vi "2 station_keeping_points.vi"(9 "Which Point?":i32, 10 "Midpoint":T1 {"North" format="%#_10f"; "East" format="%#_8f"}) -> (2 "Waypoint":T1 {"North" format="%#_10f"; "East" format="%#_8f"})   [LabVIEW 2011]
doc: "The station keeping mission steps through a series of waypoints from 1 : n. This takes which point it is on, and returns the coordinates. It uses modular arithmetic to cycle through a set of waypoints. The waypoints are shifted upwind, and usually oriented with respect to the wind somehow."
uses:
  2 Typedefs/UTM Location.ctl
  2 Typedefs/absolute wind direction.ctl
  2 Globals/2 Global.vi
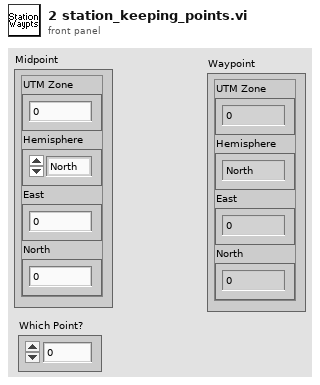
[diagram p1: front panel]
types:
  T1 = typedef "UTM Location.ctl" = cluster{"UTM Zone":i32, "Hemisphere":enum16{"North", "South"}, "East":dbl, "North":dbl}
  T2 = typedef "absolute wind direction.ctl" = dbl
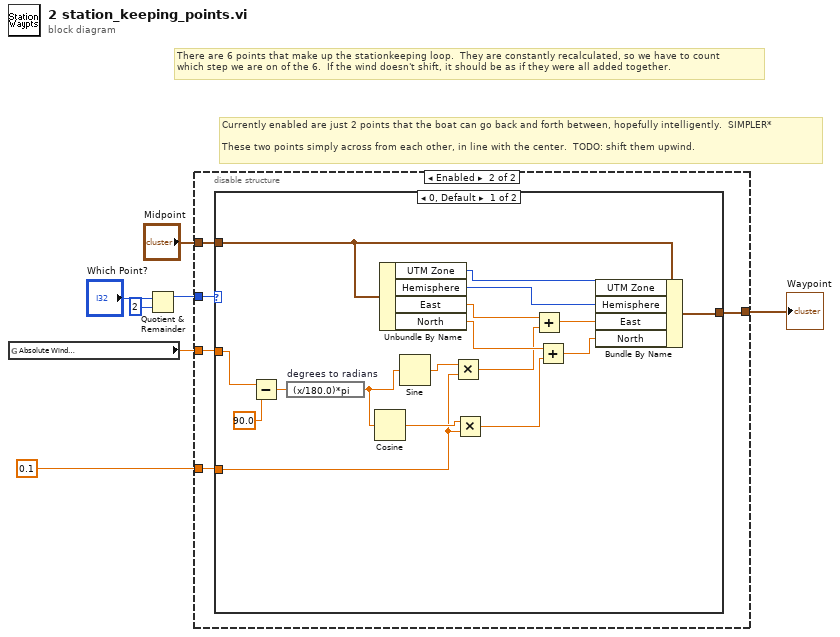
[diagram p0: block diagram]
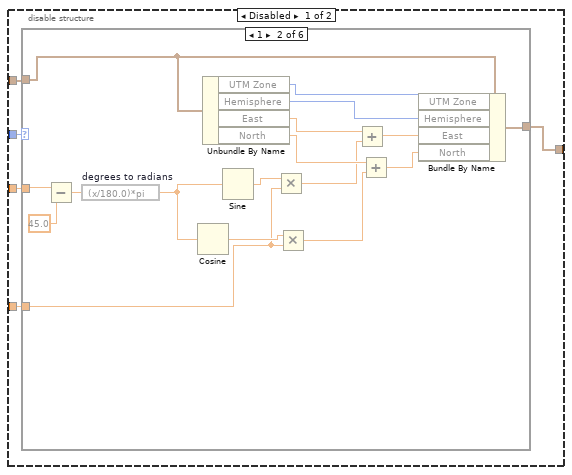
[diagram p2: hidden frame]
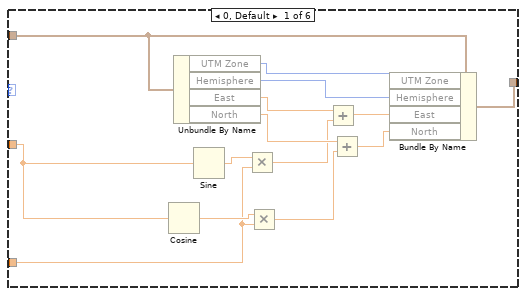
[diagram p3: hidden frame]
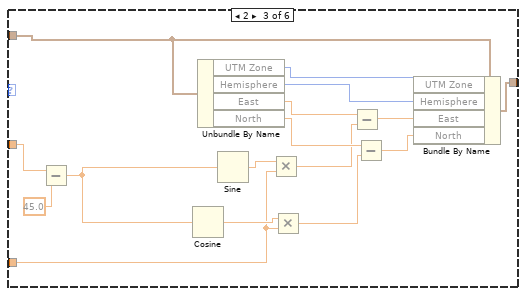
[diagram p4: hidden frame]
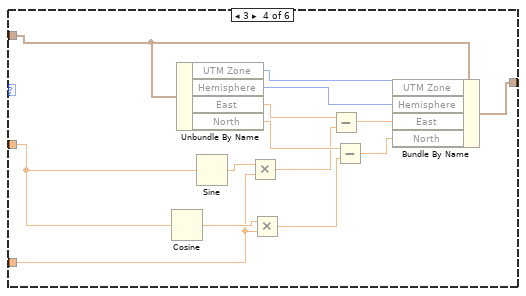
[diagram p5: hidden frame]
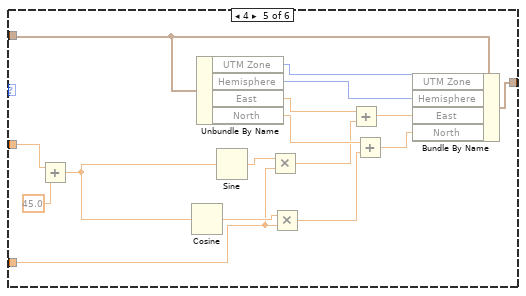
[diagram p6: hidden frame]
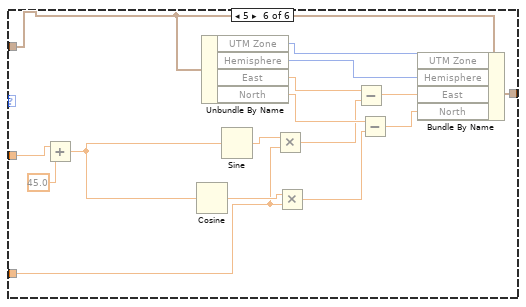
[diagram p7: hidden frame]
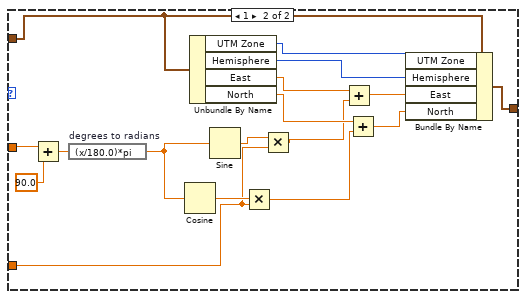
[diagram p8: hidden frame]
diagram:
  # "Currently enabled are just 2 points that the boat can go back and forth between, hopefully intelligently.  SIMPLER*\n\nThese two points simply across from each other, in line with the center.  TODO: shift them upwind."
  # "There are 6 points that make up the stationkeeping loop.  They are constantly recalculated, so we have to count\nwhich step we are on of the 6.  If the wind doesn't shift, it should be as if they were all added together."
  n1 = global read "2 Global.vi" "Absolute Wind\nDirection (º)"() -> (w3:T2)
  n2 = Quotient & Remainder(x="Which Point?", y=2) -> (x-y*floor(x/y)=w5:i32)  [unwired: 1 out]
  n3 = disable-structure shown="Enabled" {
    disable-tunnel: w5 -> [w12 w110]
    disable-tunnel: "Midpoint" -> [w11 w109]
    disable-tunnel: w3 -> [w10 w108]
    disable-tunnel: [w9 w106] -> w2
    disable-tunnel: T2 0.1 ("y") -> [w8 w107]
    frame Disabled {
      n4 = case shown="1" w12 {
        tunnel: w11 -> [w25 w32 w46 w62 w76 w92]
        tunnel: w10 -> [w14 w31 w45 w61 w75 w91]
        tunnel: [w26 w33 w47 w63 w77 w93] -> w9
        tunnel: w8 -> [w13 w29 w44 w60 w74 w90]
        frame 0, Default {
          n5 = Cosine(x=w14) -> (cos(x)=w21:T2)
          n6 = Unbundle By Name(w25) -> ("UTM Zone"=w24:i32, "Hemisphere"=w23:enum16{"North", "South"}, "East"=w19:dbl, "North"=w17:dbl)
          n7 = Sine(x=w14) -> (sin(x)=w22:T2)
          n8 = Multiply(x=w22, y=w13) -> (x*y=w16:T2)
          n9 = Multiply(x=w21, y=w13) -> (x*y=w15:T2)
          n10 = Add(x=w19, y=w16) -> (x+y=w20:T2)
          n11 = Add(x=w17, y=w15) -> (x+y=w18:T2)
          n12 = Bundle By Name(cluster=w25, "UTM Zone"=w24, "Hemisphere"=w23, "East"=w20, "North"=w18) -> (w26:T1)
        }
        frame 1 {
          n13 = Subtract(x=w31, y=T2 45.0) -> (x-y=w28:T2)
          n14 = expression code="(x/180.0)*pi" "degrees to radians"(w28) -> (w27:T2)
          n15 = Cosine(x=w27) -> (cos(x)=w40:T2)
          n16 = Unbundle By Name(w32) -> ("UTM Zone"=w43:i32, "Hemisphere"=w42:enum16{"North", "South"}, "East"=w38:dbl, "North"=w36:dbl)
          n17 = Sine(x=w27) -> (sin(x)=w41:T2)
          n18 = Multiply(x=w41, y=w29) -> (x*y=w35:T2)
          n19 = Multiply(x=w40, y=w29) -> (x*y=w34:T2)
          n20 = Add(x=w38, y=w35) -> (x+y=w39:T2)
          n21 = Add(x=w36, y=w34) -> (x+y=w37:T2)
          n22 = Bundle By Name(cluster=w32, "UTM Zone"=w43, "Hemisphere"=w42, "East"=w39, "North"=w37) -> (w33:T1)
        }
        frame 2 {
          n23 = Subtract(x=w45, y=T2 45.0) -> (x-y=w49:T2)
          n24 = Cosine(x=w49) -> (cos(x)=w56:T2)
          n25 = Unbundle By Name(w46) -> ("UTM Zone"=w59:i32, "Hemisphere"=w58:enum16{"North", "South"}, "East"=w54:dbl, "North"=w52:dbl)
          n26 = Sine(x=w49) -> (sin(x)=w57:T2)
          n27 = Multiply(x=w57, y=w44) -> (x*y=w51:T2)
          n28 = Multiply(x=w56, y=w44) -> (x*y=w50:T2)
          n29 = Subtract(x=w54, y=w51) -> (x-y=w55:T2)
          n30 = Subtract(x=w52, y=w50) -> (x-y=w53:T2)
          n31 = Bundle By Name(cluster=w46, "UTM Zone"=w59, "Hemisphere"=w58, "East"=w55, "North"=w53) -> (w47:T1)
        }
        frame 3 {
          n32 = Cosine(x=w61) -> (cos(x)=w70:T2)
          n33 = Unbundle By Name(w62) -> ("UTM Zone"=w73:i32, "Hemisphere"=w72:enum16{"North", "South"}, "East"=w68:dbl, "North"=w66:dbl)
          n34 = Sine(x=w61) -> (sin(x)=w71:T2)
          n35 = Multiply(x=w71, y=w60) -> (x*y=w65:T2)
          n36 = Multiply(x=w70, y=w60) -> (x*y=w64:T2)
          n37 = Subtract(x=w68, y=w65) -> (x-y=w69:T2)
          n38 = Subtract(x=w66, y=w64) -> (x-y=w67:T2)
          n39 = Bundle By Name(cluster=w62, "UTM Zone"=w73, "Hemisphere"=w72, "East"=w69, "North"=w67) -> (w63:T1)
        }
        frame 4 {
          n40 = Add(x=w75, y=T2 45.0) -> (x+y=w79:T2)
          n41 = Cosine(x=w79) -> (cos(x)=w86:T2)
          n42 = Unbundle By Name(w76) -> ("UTM Zone"=w89:i32, "Hemisphere"=w88:enum16{"North", "South"}, "East"=w84:dbl, "North"=w82:dbl)
          n43 = Sine(x=w79) -> (sin(x)=w87:T2)
          n44 = Multiply(x=w87, y=w74) -> (x*y=w81:T2)
          n45 = Multiply(x=w86, y=w74) -> (x*y=w80:T2)
          n46 = Add(x=w84, y=w81) -> (x+y=w85:T2)
          n47 = Add(x=w82, y=w80) -> (x+y=w83:T2)
          n48 = Bundle By Name(cluster=w76, "UTM Zone"=w89, "Hemisphere"=w88, "East"=w85, "North"=w83) -> (w77:T1)
        }
        frame 5 {
          n49 = Add(x=w91, y=T2 45.0) -> (x+y=w95:T2)
          n50 = Cosine(x=w95) -> (cos(x)=w102:T2)
          n51 = Unbundle By Name(w92) -> ("UTM Zone"=w105:i32, "Hemisphere"=w104:enum16{"North", "South"}, "East"=w100:dbl, "North"=w98:dbl)
          n52 = Sine(x=w95) -> (sin(x)=w103:T2)
          n53 = Multiply(x=w103, y=w90) -> (x*y=w97:T2)
          n54 = Multiply(x=w102, y=w90) -> (x*y=w96:T2)
          n55 = Subtract(x=w100, y=w97) -> (x-y=w101:T2)
          n56 = Subtract(x=w98, y=w96) -> (x-y=w99:T2)
          n57 = Bundle By Name(cluster=w92, "UTM Zone"=w105, "Hemisphere"=w104, "East"=w101, "North"=w99) -> (w93:T1)
        }
      }
    }
    frame Enabled {
      n58 = case shown="0, Default" w110 {
        tunnel: w109 -> [w126 w134]
        tunnel: w108 -> [w112 w133]
        tunnel: [w127 w135] -> w106
        tunnel: w107 -> [w115 w131]
        frame 0, Default {
          n59 = Subtract(x=w112, y=T2 90.0) -> (x-y=w113:T2)
          n60 = expression code="(x/180.0)*pi" "degrees to radians"(w113) -> (w111:T2)
          n61 = Cosine(x=w111) -> (cos(x)=w122:T2)
          n62 = Unbundle By Name(w126) -> ("UTM Zone"=w125:i32, "Hemisphere"=w124:enum16{"North", "South"}, "East"=w120:dbl, "North"=w118:dbl)
          n63 = Sine(x=w111) -> (sin(x)=w123:T2)
          n64 = Multiply(x=w123, y=w115) -> (x*y=w117:T2)
          n65 = Multiply(x=w122, y=w115) -> (x*y=w116:T2)
          n66 = Add(x=w120, y=w117) -> (x+y=w121:T2)
          n67 = Add(x=w118, y=w116) -> (x+y=w119:T2)
          n68 = Bundle By Name(cluster=w126, "UTM Zone"=w125, "Hemisphere"=w124, "East"=w121, "North"=w119) -> (w127:T1)
        }
        frame 1 {
          n69 = Add(x=w133, y=T2 90.0) -> (x+y=w130:T2)
          n70 = expression code="(x/180.0)*pi" "degrees to radians"(w130) -> (w129:T2)
          n71 = Cosine(x=w129) -> (cos(x)=w141:T2)
          n72 = Unbundle By Name(w134) -> ("UTM Zone"=w144:i32, "Hemisphere"=w143:enum16{"North", "South"}, "East"=w139:dbl, "North"=w137:dbl)
          n73 = Sine(x=w129) -> (sin(x)=w142:T2)
          n74 = Multiply(x=w141, y=w131) -> (x*y=w136:T2)
          n75 = Multiply(x=w142, y=w131) -> (x*y=w128:T2)
          n76 = Add(x=w139, y=w128) -> (x+y=w140:T2)
          n77 = Add(x=w137, y=w136) -> (x+y=w138:T2)
          n78 = Bundle By Name(cluster=w134, "UTM Zone"=w144, "Hemisphere"=w143, "East"=w140, "North"=w138) -> (w135:T1)
        }
      }
    }
  }
  "Waypoint" <- w2
